vi "WSVCAP SHL Host LL Remap DUT and Socket Locations.vi"(0 "C1 DUT Ordered Data In":u8[][](array[numeric]) format="%.0x", 1 "C2 DUT Ordered Data In":u8[][](array[numeric]) format="%.0x", 2 "C3 DUT Ordered Data In":u8[][](array[numeric]) format="%.0x", 3 "C1 Socket Ordered Data In":u8[][](array[numeric]) format="%.0x", 4 "C2 Socket Ordered Data In":u8[][](array[numeric]) format="%.0x", 5 "C3 Socket Ordered Data In":u8[][](array[numeric]) format="%.0x") -> (14 "C1 Socket Ordered Data Out":u8[][](array[numeric]) format="%.0x", 15 "C2 Socket Ordered Data Out":u8[][](array[numeric]) format="%.0x", 16 "C3 Socket Ordered Data Out":u8[][](array[numeric]) format="%.0x", 17 "C1 DUT Ordered Data Out":u8[][](array[numeric]) format="%.0x", 18 "C2 DUT Ordered Data Out":u8[][](array[numeric]) format="%.0x", 19 "C3 DUT Ordered Data Out":u8[][](array[numeric]) format="%.0x")   [LabVIEW 2012]
uses:
  Type Defs/WSVCAP SHL DUT Number Enum.ctl
panel:
  out "DUT/SOCKET Map":string[](array[string])=["DUT 01 [S08-H]", "DUT 02 [S07-G]", "DUT 03 [S09-I]", "DUT 04 [S10-J]", "DUT 05 [S06-F]", "DUT 06 [S05-E]", "DUT 07 [S12-L]", "DUT 08 [S11-K]", "DUT 09 [S03-C]", "DUT 10 [S04-D]", "DUT 11 [S13-M]", "DUT 12 [S14-N]", "DUT 13 [S02-B]", "DUT 14 [S01-A]", "DUT 15 [S16-P]", "DUT 16 [S15-O]"]
  in  "DUT Number":T1
  # "DUT 01"
  # "DUT 02"
  # "DUT 03"
  # "DUT 04"
  # "DUT 05"
  # "DUT 06"
  # "DUT 07"
  # "DUT 08"
  # "DUT 09"
  # "DUT 10"
  # "DUT 11"
  # "DUT 12"
  # "DUT 13"
  # "DUT 14"
  # "DUT 15"
  # "DUT 16"
  # "SKT 01"
  # "SKT 02"
  # "SKT 03"
  # "SKT 04"
  # "SKT 05"
  # "SKT 06"
  # "SKT 07"
  # "SKT 08"
  # "SKT 09"
  # "SKT 10"
  # "SKT 11"
  # "SKT 12"
  # "SKT 13"
  # "SKT 14"
  # "SKT 15"
  # "SKT 16"
  # "DUT 01"
  # "DUT 02"
  # "DUT 03"
  # "DUT 04"
  # "DUT 05"
  # "DUT 06"
  # "DUT 07"
  # "DUT 08"
  # "DUT 09"
  # "DUT 10"
  # "DUT 11"
  # "DUT 12"
  # "DUT 13"
  # "DUT 14"
  # "DUT 15"
  # "DUT 16"
  # "SKT 01"
  # "SKT 02"
  # "SKT 03"
  # "SKT 04"
  # "SKT 05"
  # "SKT 06"
  # "SKT 07"
  # "SKT 08"
  # "SKT 09"
  # "SKT 10"
  # "SKT 11"
  # "SKT 12"
  # "SKT 13"
  # "SKT 14"
  # "SKT 15"
  # "SKT 16"
  # "DUT 01"
  # "DUT 02"
  # "DUT 03"
  # "DUT 04"
  # "DUT 05"
  # "DUT 06"
  # "DUT 07"
  # "DUT 08"
  # "DUT 09"
  # "DUT 10"
  # "DUT 11"
  # "DUT 12"
  # "DUT 13"
  # "DUT 14"
  # "DUT 15"
  # "DUT 16"
  # "SKT 01"
  # "SKT 02"
  # "SKT 03"
  # "SKT 04"
  # "SKT 05"
  # "SKT 06"
  # "SKT 07"
  # "SKT 08"
  # "SKT 09"
  # "SKT 10"
  # "SKT 11"
  # "SKT 12"
  # "SKT 13"
  # "SKT 14"
  # "SKT 15"
  # "SKT 16"
  # "DUT 01"
  # "DUT 02"
  # "DUT 03"
  # "DUT 04"
  # "DUT 05"
  # "DUT 06"
  # "DUT 07"
  # "DUT 08"
  # "DUT 09"
  # "DUT 10"
  # "DUT 11"
  # "DUT 12"
  # "DUT 13"
  # "DUT 14"
  # "DUT 15"
  # "DUT 16"
  # "SKT 01"
  # "SKT 02"
  # "SKT 03"
  # "SKT 04"
  # "SKT 05"
  # "SKT 06"
  # "SKT 07"
  # "SKT 08"
  # "SKT 09"
  # "SKT 10"
  # "SKT 11"
  # "SKT 12"
  # "SKT 13"
  # "SKT 14"
  # "SKT 15"
  # "SKT 16"
  # "DUT 01"
  # "DUT 02"
  # "DUT 03"
  # "DUT 04"
  # "DUT 05"
  # "DUT 06"
  # "DUT 07"
  # "DUT 08"
  # "DUT 09"
  # "DUT 10"
  # "DUT 11"
  # "DUT 12"
  # "DUT 13"
  # "DUT 14"
  # "DUT 15"
  # "DUT 16"
  # "SKT 01"
  # "SKT 02"
  # "SKT 03"
  # "SKT 04"
  # "SKT 05"
  # "SKT 06"
  # "SKT 07"
  # "SKT 08"
  # "SKT 09"
  # "SKT 10"
  # "SKT 11"
  # "SKT 12"
  # "SKT 13"
  # "SKT 14"
  # "SKT 15"
  # "SKT 16"
  # "SKT 01"
  # "SKT 02"
  # "SKT 03"
  # "SKT 04"
  # "SKT 05"
  # "SKT 06"
  # "SKT 07"
  # "SKT 08"
  # "SKT 09"
  # "SKT 10"
  # "SKT 11"
  # "SKT 12"
  # "SKT 13"
  # "SKT 14"
  # "SKT 15"
  # "SKT 16"
  # "DUT 01"
  # "DUT 02"
  # "DUT 03"
  # "DUT 04"
  # "DUT 05"
  # "DUT 06"
  # "DUT 07"
  # "DUT 08"
  # "DUT 09"
  # "DUT 10"
  # "DUT 11"
  # "DUT 12"
  # "DUT 13"
  # "DUT 14"
  # "DUT 15"
  # "DUT 16"
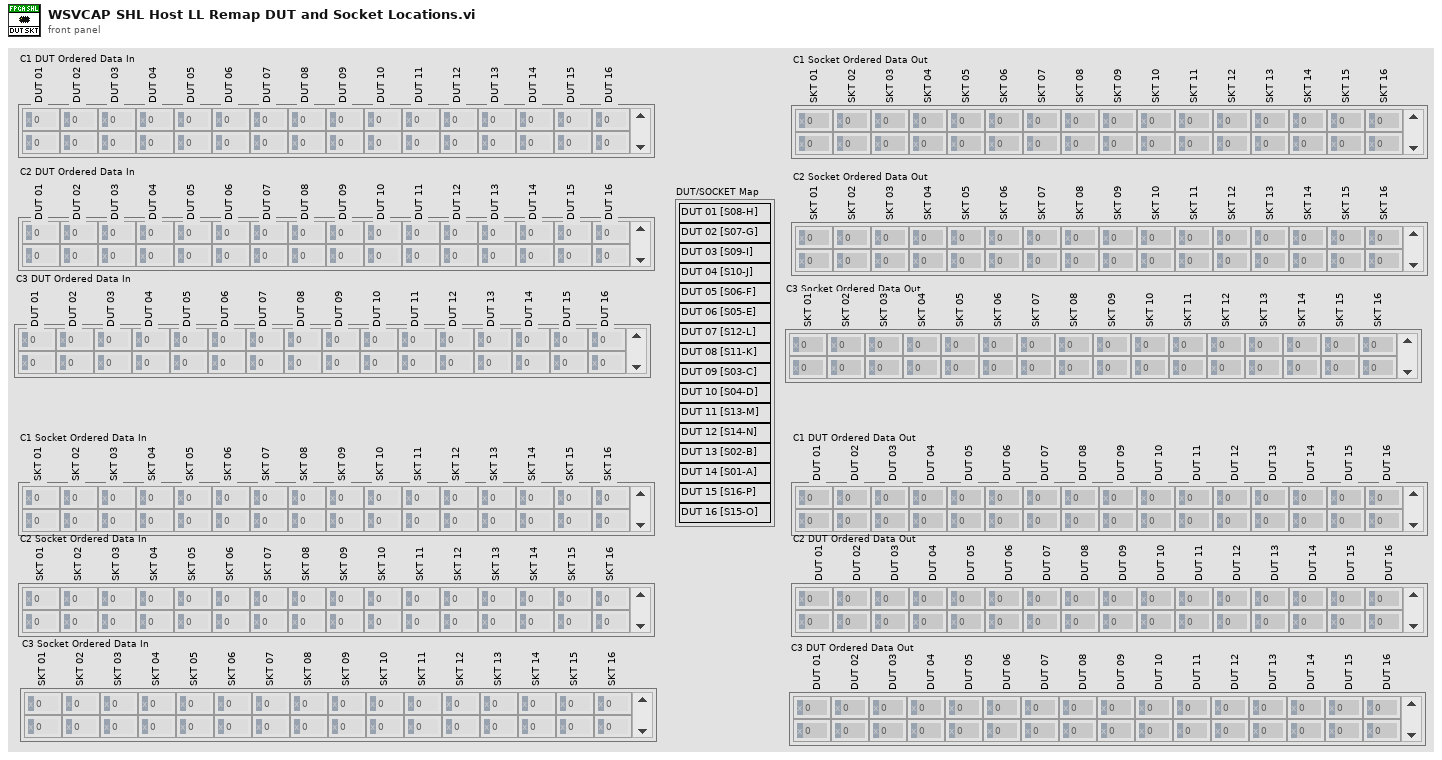
[diagram p1: front panel]
types:
  T1 = typedef "WSVCAP SHL DUT Number Enum.ctl" = enum16{"DUT 01 [S01-A]", "DUT 02 [S02-B]", "DUT 03 [S03-C]", "DUT 04 [S04-D]", "DUT 05 [S05-E]", "DUT 06 [S06-F]", "DUT 07 [S07-G]", "DUT 08 [S08-H]", "DUT 09 [S09-I]", "DUT 10 [S10-J]", "DUT 11 [S11-K]", "DUT 12 [S12-L]", "DUT 13 [S13-M]", "DUT 14 [S14-N]", "DUT 15 [S15-O]", "DUT 16 [S16-P]"}
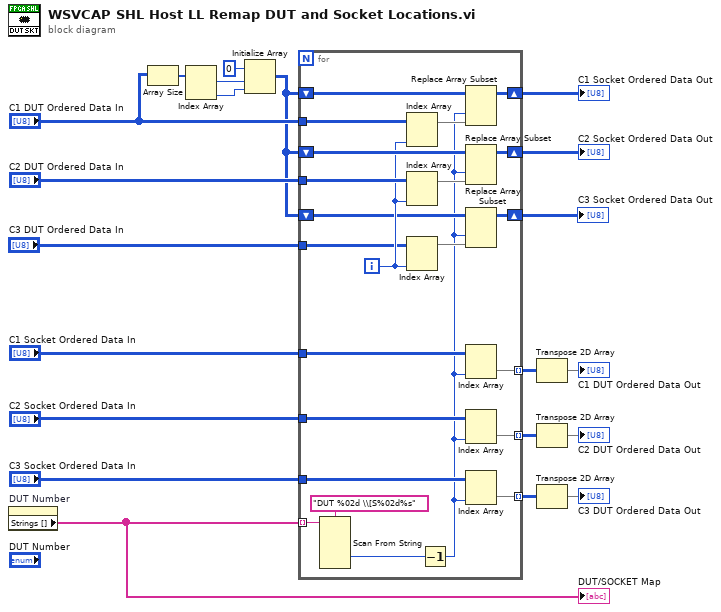
[diagram p0: block diagram]
diagram:
  n1 = property on="DUT Number" class="Enum (strict)"() -> ("Strings []"=w12:string[])  [unwired: 2 in, 2 out]
  "DUT/SOCKET Map" <- w12
  n2 = Array Size(array="C1 DUT Ordered Data In") -> (size(s)=w10:i32[])
  n3 = Index Array(array=w10) -> (element #1=w9:i32, element #2=w8:i32)  [unwired: 2 in]
  n4 = Initialize Array(u8 0 ("element"), w9, w8) -> (w5:u8[][])
  n5 = for {
    tunnel: w12 -> [w42] mode=indexing
    tunnel: "C1 DUT Ordered Data In" -> [w44]
    tunnel: "C1 Socket Ordered Data In" -> [w41]
    tunnel: [w40] -> w20 mode=indexing
    shift-right: [w38] -> w18
    shift-left: w5 -> [w39]
    shift-right: [w33] -> w16
    shift-left: w5 -> [w34]
    tunnel: "C2 DUT Ordered Data In" -> [w32]
    tunnel: "C2 Socket Ordered Data In" -> [w31]
    tunnel: [w30] -> w14 mode=indexing
    tunnel: "C3 DUT Ordered Data In" -> [w28]
    shift-right: [w26] -> w4
    shift-left: w5 -> [w27]
    tunnel: [w24] -> w3 mode=indexing
    tunnel: "C3 Socket Ordered Data In" -> [w23]
    i -> [w29]
    n6 = Scan From String(format string="DUT %02d \\[S%02d%s", input string=w42) -> (output 2=w37:i32)  [unwired: 7 in, 3 out]
    n7 = Index Array(array=w44, index (col)=w29) -> (element=w36:u8[])  [unwired: 1 in]
    n8 = Index Array(array=w32, index (col)=w29) -> (element=w35:u8[])  [unwired: 1 in]
    n9 = Index Array(array=w28, index (col)=w29) -> (element=w25:u8[])  [unwired: 1 in]
    n10 = Decrement(x=w37) -> (x-1=w22:i32)
    n11 = Replace Array Subset(array=w39, new element=w36, index (col)=w22) -> (w38:u8[][])  [unwired: 1 in]
    n12 = Replace Array Subset(array=w34, new element=w35, index (col)=w22) -> (w33:u8[][])  [unwired: 1 in]
    n13 = Replace Array Subset(array=w27, new element=w25, index (col)=w22) -> (w26:u8[][])  [unwired: 1 in]
    n14 = Index Array(array=w41, index (col)=w22) -> (element=w40:u8[])  [unwired: 1 in]
    n15 = Index Array(array=w31, index (col)=w22) -> (element=w30:u8[])  [unwired: 1 in]
    n16 = Index Array(array=w23, index (col)=w22) -> (element=w24:u8[])  [unwired: 1 in]
  }
  "C1 Socket Ordered Data Out" <- w18
  "C2 Socket Ordered Data Out" <- w16
  "C3 Socket Ordered Data Out" <- w4
  n17 = Transpose 2D Array(2D array=w20) -> (transposed array=→"C1 DUT Ordered Data Out":u8[][])
  n18 = Transpose 2D Array(2D array=w14) -> (transposed array=→"C2 DUT Ordered Data Out":u8[][])
  n19 = Transpose 2D Array(2D array=w3) -> (transposed array=→"C3 DUT Ordered Data Out":u8[][])
